vi "WritePersistentConfiguration.vi"(8 "ErrorIn":errorcluster, 10 "DataIn":variant, 11 "TemplateGUITAFIn":refnum<class "TemplateGUITAF.lvclass">) -> (0 "ErrorOut":errorcluster, 2 "DataOut":variant, 3 "TemplateGUITAFOut":refnum<class "TemplateGUITAF.lvclass">)   [LabVIEW 2021, in "TemplateGUITAF.lvlib" / "TemplateGUITAF.lvclass"]
uses:
  TemplateGUITAF.lvclass
  TemplateGUITAF.lvclass/TemplateGUITAF.ctl
  907f2fb5-1632-40ed-9d2f-4bf6232f9664.vi
  <vilib>/Utility/LVClass/Get LV Class Name.vi
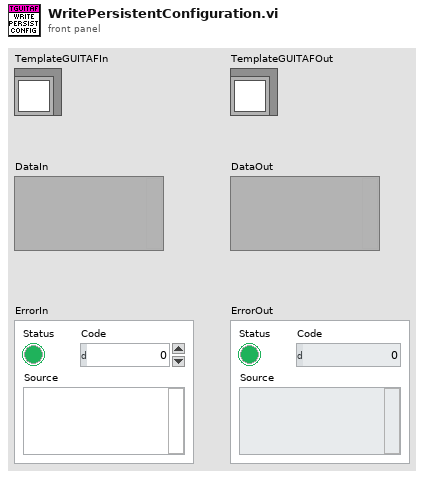
[diagram p1: front panel]
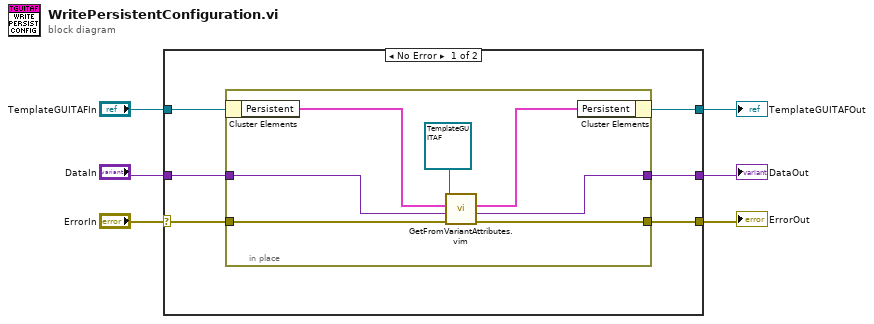
[diagram p0: block diagram]
diagram:
  n1 = case shown="No Error" "ErrorIn" {
    selector: "ErrorIn" -> [w12 w22]
    tunnel: [w11 w22] -> w5
    tunnel: [w10 w21] -> w3
    tunnel: "TemplateGUITAFIn" -> [w9 w21]
    tunnel: "DataIn" -> [w8 w20]
    tunnel: [w7 w20] -> w1
    frame No Error {
      n2 = in-place {
        in-place-border: [w19] -> w11
        in-place-border: w8 -> [w17]
        in-place-border: [w16] -> w7
        in-place-border: w12 -> [w18]
        n3 = in-place-cluster #1(w9) -> ("Persistent"=w15:cluster{"dummy":bool})
        n4 = call "GetFromVariantAttributes.vim"("ErrorIn"=w18, "DataInIn"=w17, "PersistentDataType"=w15, "Object"=refnum<class "TemplateGUITAF.lvclass"> refnum ("ApplicationGUI2")) -> ("ErrorOut"=w19:errorcluster, "DataOut"=w16:variant, "PersistentDataOut"=w14:cluster{"dummy":bool})  [unwired: 5 in]
        n5 = in-place-cluster #1("Persistent"=w14) -> (w10:refnum<class "TemplateGUITAF.lvclass">)
      }
    }
    frame Error {
    }
  }
  "ErrorOut" <- w5
  "TemplateGUITAFOut" <- w3
  "DataOut" <- w1
